vi "libdaq_init.vi"(0 "error in (no error)":errorcluster) -> (14 "error out":errorcluster)   [LabVIEW 2010, in "libdaqVI.lvlib"]
doc: "libdaq库初始化，该函数必须在调用任何其他API之前调用，见库初始化章节"
uses:
  libdaqVI.lvlib
  dll/daqlib.dll
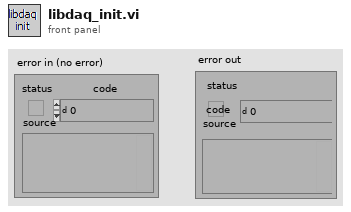
[diagram p1: front panel]
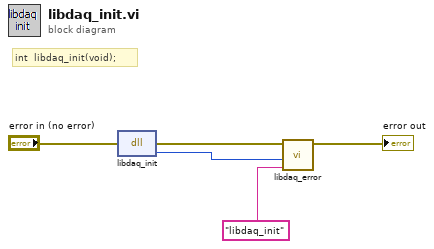
[diagram p0: block diagram]
diagram:
  # "int  libdaq_init(void);"
  n1 = dll-call lib="E:/Product/Example/DAQ-USB3212/Labview/labview_2010/libdaqVI/dll/daqlib.dll" fn="libdaq_init"(error in="error in (no error)") -> (error out=w4:errorcluster, "return type"=w2:i32)  [unwired: 2 in, 1 out]
  n2 = call "libdaq_error.vi"("error source"="libdaq_init", "error code"=w2, "错误输入（无错误）"=w4) -> ("错误输出"=→"error out":errorcluster)  [unwired: 8 in]
